vi "Cpci_Read.vi"(8 "错误输入（无错误）":errorcluster, 9 "u32_len":i32, 10 "基地址":u32=1048576 format="%.0x", 11 "VISA资源名称":refnum<visa-resource-name>) -> (0 "错误输出":errorcluster, 2 "U8":u8[](array[numeric]), 3 "VISA资源名称输出":refnum<visa-resource-name>)   [LabVIEW 2012]
uses:
  <vilib>/Instr/_visa.llb/VISA Register Access Address Space.ctl
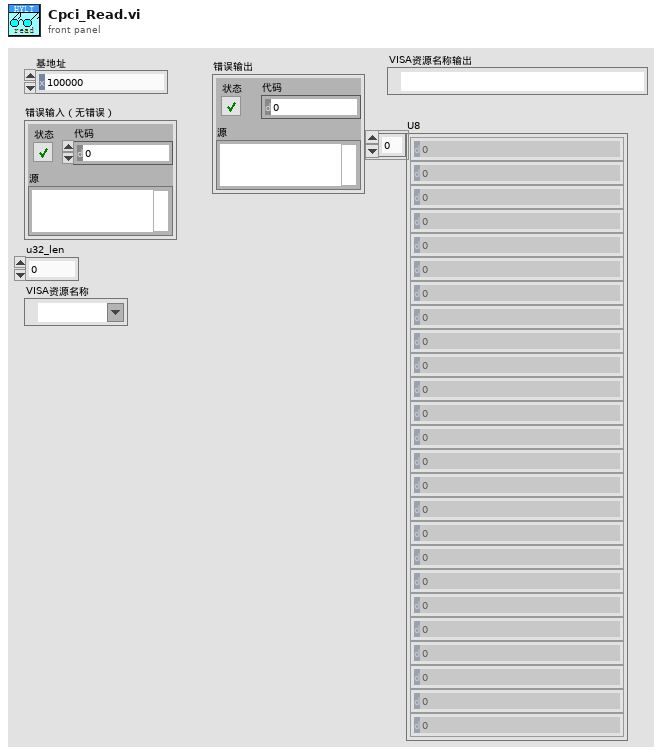
[diagram p1: front panel]
types:
  T1 = typedef "VISA Register Access Address Space.ctl" = u16
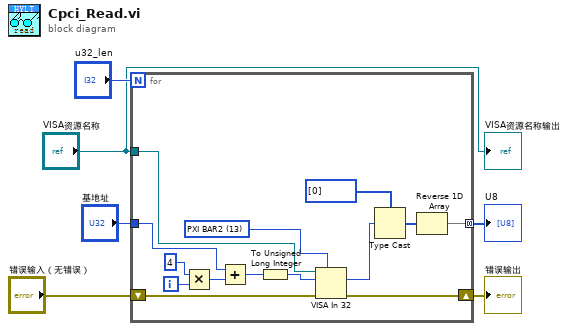
[diagram p0: block diagram]
diagram:
  n1 = for {
    N: "u32_len" -> [_]
    tunnel: "基地址" -> [w17]
    tunnel: "VISA资源名称" -> [w16]
    shift-right: [w7] -> w2
    shift-left: "错误输入（无错误）" -> [w14]
    tunnel: [w8] -> w3 mode=concatenating
    i -> [w19]
    w15 = T1 13 items=["VXI/VME A16"=1, "VXI/VME A24"=2, "VXI/VME A32"=3, "VXI/VME A64"=4, "PXI内存分配"=9, "PXI配置"=10, "PXI BAR0"=11, "PXI BAR1"=12, "PXI BAR2"=13, "PXI BAR3"=14, "PXI BAR4"=15, "PXI BAR5"=16] ("Address Space")
    n2 = Multiply(x=4, y=w19) -> (x*y=w20:i32)
    n3 = Add(x=w17, y=w20) -> (x+y=w13:u32)
    n4 = To Unsigned Long Integer(number=w13) -> (unsigned 32bit integer=w12:u32)
    n5 = VISA In 32(7:w15, 8:w14, 10:w12, 11:w16) -> (0:w7:errorcluster, 2:w9:u32)  [unwired: 1 out]
    n6 = Type Cast(type=u8[] [0], x=w9) -> (*(type *) &x=w11:u8[])
    n7 = Reverse 1D Array(array=w11) -> (reversed array=w8:u8[])
  }
  "错误输出" <- w2
  "U8" <- w3
  "VISA资源名称输出" <- "VISA资源名称"
